vi "P2Y1.vi"() -> ()   [LabVIEW 2020]
panel:
  in  "Slide":dbl(slide) scale=-100.0..100.0
  in  "stop":bool
  out "Waveform Chart":dbl(graph)
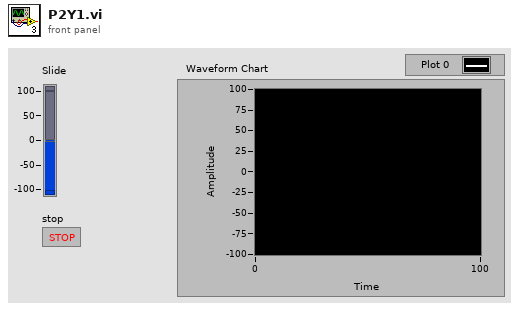
[diagram p1: front panel]
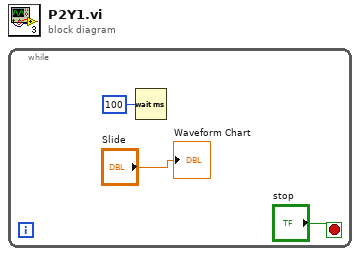
[diagram p0: block diagram]
diagram:
  n1 = while {
    stop <- "stop" stop-if-true
    n2 = Wait (ms)(milliseconds to wait=u32 100) -> ()  [unwired: 1 out]
    "Waveform Chart" <- "Slide"
  }
